vi "判断指定文件里有否 需要的EXCEL文档   如果没有就从模板文件里复制一个过去 然后改名字 最后  修改名字后EXCEL文档的路径.vi"(2 "输入参数三：错误输入":errorcluster, 3 "参数二：目标文件夹，就是被罗列的文件夹的路径":path, 4 "参数一：这里面放置被复制的模板文件":path) -> (0 "输出参数二：错误输出":errorcluster, 1 "输出参数一：修改完名字的路径":path)   [LabVIEW 2014]
panel:
  # "工控机和上位软件讨论：20423623  主题：讨论上位系统：WINCC LABVIEW  INTOUCH MATLAB VB VC \n\n电气制图软件交流促进：182667049  主题：EPLAN  CAD PCSCHEMATIC 等\n\n电子学习共同促进群：234742235   主题：学习探讨单片机 电子线路等电子技术\n\n自动化行业非标PLC编程：170665069     主题：坦诚沟通 共同进步\n\n运动控制机器人视觉 : 254438239主题：运动控制卡：英国翠欧，美国PMAC，英国BALDOR  机器人：ABB 爱普生 三菱 雅马哈 CCD"
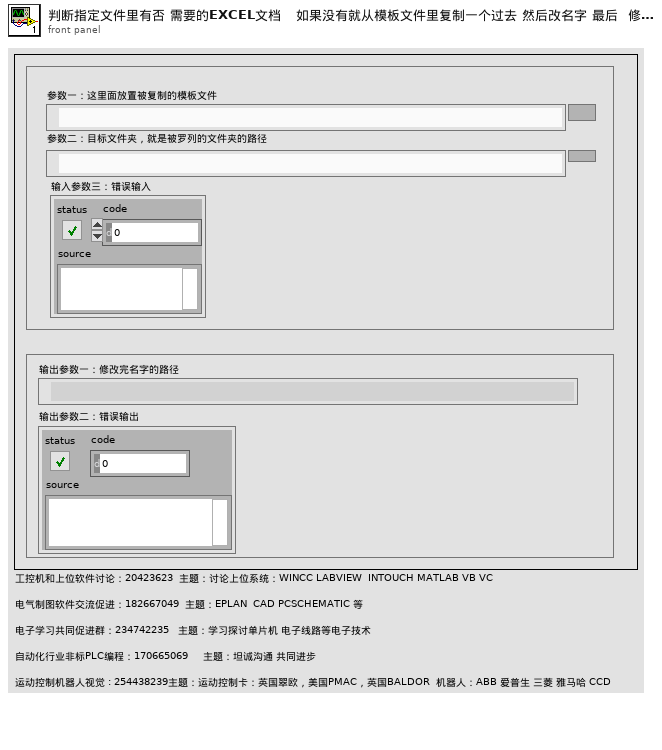
[diagram p1: front panel]
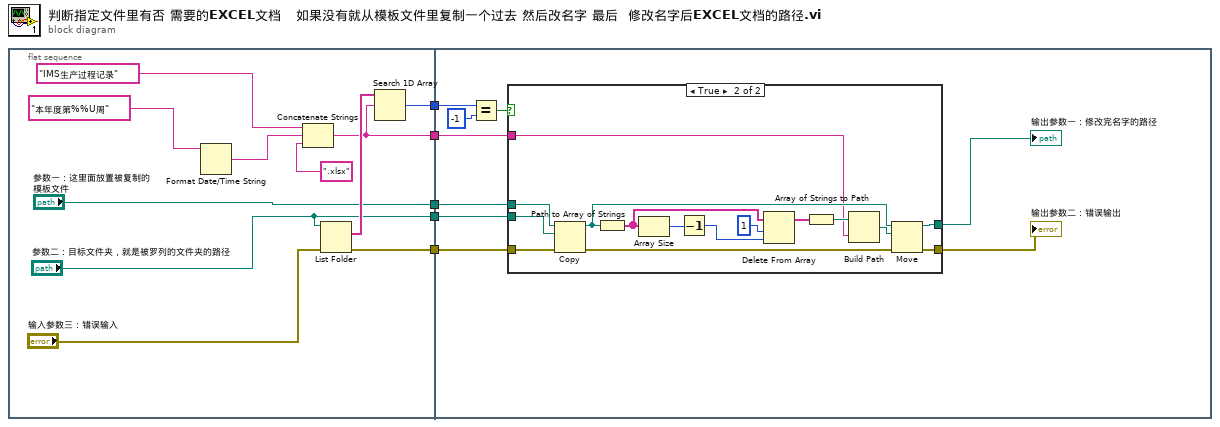
[diagram p0: block diagram]
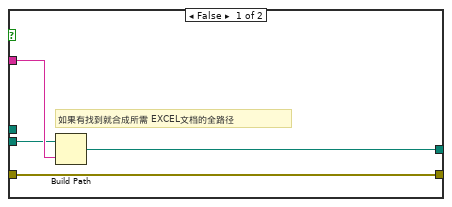
[diagram p2: hidden frame]
diagram:
  n1 = flat-sequence {
    tunnel: [w10] -> w5
    tunnel: [w9] -> w4
    tunnel: ["参数二：目标文件夹，就是被罗列的文件夹的路径"] -> w3
    tunnel: [w7] -> w2
    tunnel: ["参数一：这里面放置被复制的模板文件"] -> w1
    tunnel: w5 -> [w24]
    tunnel: w4 -> [w22]
    tunnel: w3 -> [w21]
    tunnel: w2 -> [w19]
    tunnel: w1 -> [w17]
    frame #0 {
      n2 = Format Date/Time String(time format string (%c)="本年度第%%U周") -> (date/time string=w14:string)  [unwired: 2 in]
      n3 = Concatenate Strings("IMS生产过程记录" ("string"), w14, ".xlsx" ("string")) -> (w9:string)
      n4 = List Folder(path="参数二：目标文件夹，就是被罗列的文件夹的路径", error in="输入参数三：错误输入") -> (filenames=w15:string[], error out=w7:errorcluster)  [unwired: 2 in, 2 out]
      n5 = Search 1D Array(1D array=w15, element=w9) -> (index of element=w10:i32)  [unwired: 1 in]
    }
    frame #1 {
      n6 = Equal?(x=w24, y=-1) -> (x = y?=w25:bool)
      n7 = case shown="True" w25 {
        tunnel: w22 -> [w29 w32]
        tunnel: w21 -> [w28 w34]
        tunnel: [w27 w35] -> w20
        tunnel: w19 -> [w26 w33]
        tunnel: [w26 w31] -> w18
        tunnel: w17 -> [_ w30]
        frame False {
          # "如果有找到就合成所需 EXCEL文档的全路径"
          n8 = Build Path(base path=w28, name or relative path=w29) -> (appended path=w27:path)
        }
        frame True {
          n9 = Copy(8:w33, 10:w34, 11:w30) -> (0:w44:errorcluster, 3:w36:path)  [unwired: 2 in, 1 out]
          n10 = Path to Array of Strings(0:w36) -> (2:w37:string[])  [unwired: 1 out]
          n11 = Array Size(array=w37) -> (size(s)=w42:i32)
          n12 = Decrement(x=w42) -> (x-1=w43:i32)
          n13 = Delete From Array(array=w37, length=1, index=w43) -> (array with subset deleted=w40:string[])  [unwired: 1 out]
          n14 = Array of Strings to Path(0:w40) -> (2:w39:path)  [unwired: 1 out]
          n15 = Build Path(base path=w39, name or relative path=w32) -> (appended path=w38:path)
          n16 = Move(source path=w36, error in=w44, 10:w38) -> (error out=w31:errorcluster, 3:w35:path)  [unwired: 2 in, 1 out]
        }
      }
      "输出参数一：修改完名字的路径" <- w20
      "输出参数二：错误输出" <- w18
    }
  }
